vi "Manage Save Data.vi"(8 "entrée d'erreur (pas d'erreur)":errorcluster, 10 "Data":T3(array[cluster]), 11 "Database Altyor En entrée":refnum<class "Database Altyor.lvclass">) -> (0 "sortie d'erreur":errorcluster, 3 "Database Altyor En Sortie":refnum<class "Database Altyor.lvclass">)   [LabVIEW 2020, in "Library Core.lvlib" / "Actor Test Database.lvclass"]
uses:
  Actor Test Database.lvclass
  Database/Database Altyor/Database Altyor.lvclass
  Commun VI/TypeDef/Commande Test/Commande Value Type.ctl
  Commun VI/TypeDef/Commande Test/Commande Type Test.ctl
  Actor Test Database.lvclass/Actor Test Database.ctl
  Commun VI/Library Commun.lvlib
panel:
  in  "TypeValue":T1
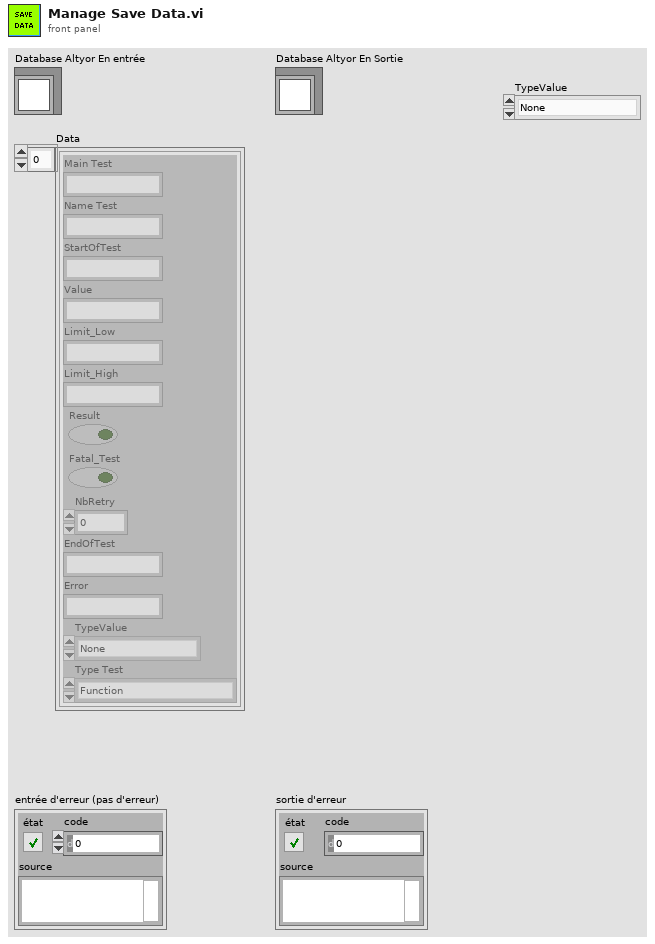
[diagram p1: front panel]
types:
  T1 = typedef "Library Commun.lvlib/Commande Value Type.ctl" = enum16{"None", "String", "Number", "Timestamp", "Boolean", "Array"}
  T2 = typedef "Library Commun.lvlib/Commande Type Test.ctl" = enum16{"Function", "Test", "Calculation"}
  T3 = cluster{"Main Test":string, "Name Test":string, "StartOfTest":string, "Value":string, "Limit_Low":string, "Limit_High":string, "Result":bool, "Fatal_Test":bool, "NbRetry":dbl, "EndOfTest":string, "Error":string, "TypeValue":T1, "Type Test":T2}[]
  T4 = cluster{"Key_Test":u32, "idTest":u32, "MainTest":string, "Name":string, "StartOfTest":string, "EndOfTest":string, "Result":string, "LimitMax":string, "Value":string, "LimitMin":string, "Type":string}
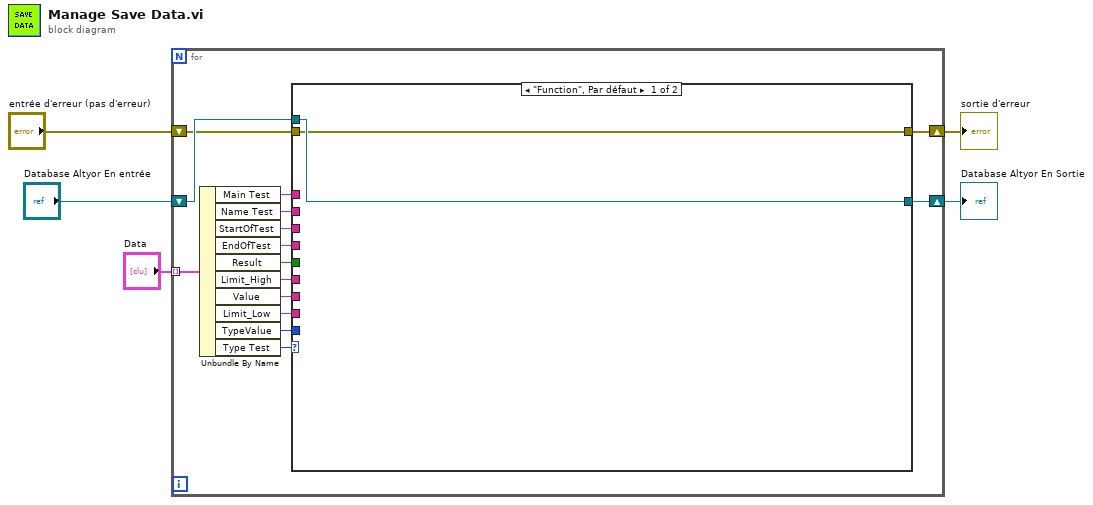
[diagram p0: block diagram]
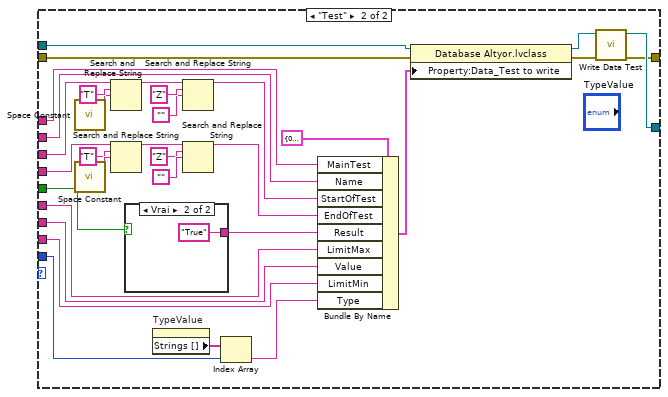
[diagram p2: hidden frame]
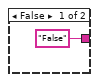
[diagram p3: hidden frame]
diagram:
  n1 = for {
    tunnel: "Data" -> [w20] mode=indexing
    shift-right: [w10] -> w3
    shift-left: "Database Altyor En entrée" -> [w12]
    shift-right: [w9] -> w1
    shift-left: "entrée d'erreur (pas d'erreur)" -> [w11]
    n2 = Unbundle By Name(w20) -> ("Main Test"=w19:string, "Name Test"=w18:string, "StartOfTest"=w8:string, "EndOfTest"=w7:string, "Result"=w14:bool, "Limit_High"=w17:string, "Value"=w16:string, "Limit_Low"=w15:string, "TypeValue"=w13:T1, "Type Test"=w6:T2)
    n3 = case shown="\"Function\", Par défaut" w6 {
      tunnel: w19 -> [_ w53]
      tunnel: w18 -> [_ w52]
      tunnel: w17 -> [_ w51]
      tunnel: w16 -> [_ w50]
      tunnel: w15 -> [_ w49]
      tunnel: w14 -> [_ w47]
      tunnel: w13 -> [_ w45]
      tunnel: w12 -> [w22 w43]
      tunnel: w11 -> [w21 w41]
      tunnel: [w22 w38] -> w10
      tunnel: [w21 w37] -> w9
      tunnel: w8 -> [_ w31]
      tunnel: w7 -> [_ w25]
      frame "Function", Default {
      }
      frame "Test" {
        n4 = call <vilib>:"Space Constant.vi"() -> ("String"=w35:string)
        n5 = call <vilib>:"Space Constant.vi"() -> ("String"=w27:string)
        n6 = Search and Replace String(input string=w31, search string="T" ("chaîne recherchée"), replace string=w35) -> (result string=w34:string)  [unwired: 5 in, 3 out]
        n7 = Search and Replace String(input string=w25, search string="T" ("chaîne recherchée"), replace string=w27) -> (result string=w28:string)  [unwired: 5 in, 3 out]
        n8 = case shown="Vrai" w47 {
          tunnel: ["False" "True"] -> w48
          frame False {
          }
          frame True {
          }
        }
        n9 = property on="TypeValue" class="Énum (strict)"() -> ("Strings []"=w46:string[])  [unwired: 2 in, 2 out]
        n10 = Search and Replace String(input string=w34, search string="Z" ("chaîne recherchée"), replace string="") -> (result string=w23:string)  [unwired: 5 in, 3 out]
        n11 = Search and Replace String(input string=w28, search string="Z" ("chaîne recherchée"), replace string="") -> (result string=w24:string)  [unwired: 5 in, 3 out]
        n12 = Index Array(array=w46, index=w45) -> (element=w44:string)
        n13 = Bundle By Name(cluster=T4 {"Key_Test"=0, "idTest"=0, "MainTest"="", "Name"="", "StartOfTest"="", "EndOfTest"="", "Result"="", "LimitMax"="", "Value"="", "LimitMin"="", "Type"=""} ("élément"), "MainTest"=w53, "Name"=w52, "StartOfTest"=w23, "EndOfTest"=w24, "Result"=w48, "LimitMax"=w51, "Value"=w50, "LimitMin"=w49, "Type"=w44) -> (w42:T4)
        n14 = property class="Database Altyor.lvclass"(reference=w43, error in=w41, "Property:Data_Test to write"=w42) -> (reference out=w39:refnum<class "Database Altyor.lvclass">, error out=w40:errorcluster)
        n15 = call-dynamic "Write Data Test.vi"("error in (no error)"=w40, "Database Altyor en entrée"=w39) -> ("error out"=w37:errorcluster, "Database Altyor en sortie"=w38:refnum<class "Database Altyor.lvclass">)  [unwired: 8 in]
      }
    }
  }
  "Database Altyor En Sortie" <- w3
  "sortie d'erreur" <- w1
